vi "RDS Serial Config.vi"(8 "error in (no error)":errorcluster, 11 "AIP Instrument in":refnum<class "AIP Instrument.lvclass">) -> (0 "error out":errorcluster, 1 "baud rate (9600)":u32, 2 "VISA resource name":refnum<visa-resource-name>, 3 "AIP Instrument out":refnum<class "AIP Instrument.lvclass">, 5 "Termination Char(s)":string)   [LabVIEW 2015]
uses:
  AIP Instrument.lvclass
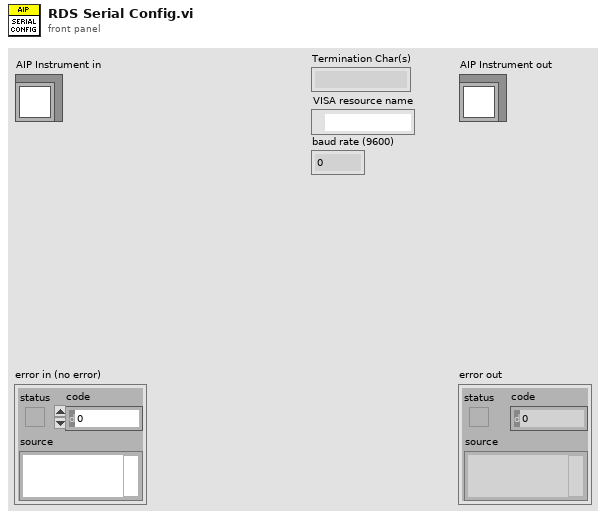
[diagram p1: front panel]
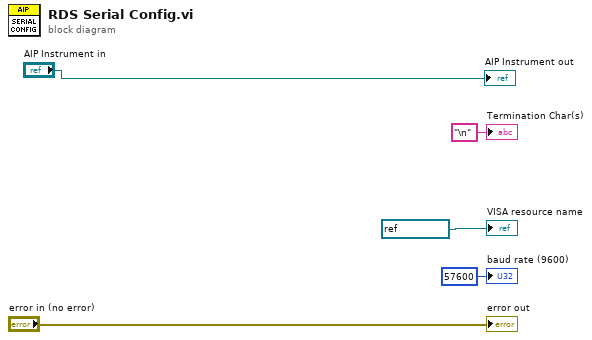
[diagram p0: block diagram]
diagram:
  "error out" <- "error in (no error)"
  "AIP Instrument out" <- "AIP Instrument in"
  "Termination Char(s)" <- "\n" ("Termination Char(s)")
  "VISA resource name" <- refnum<visa-resource-name> "COM18" ("VISA resource name")
  "baud rate (9600)" <- u32 57600 ("baud rate (9600)")
